vi "Parse_Ignore_string.vi"(0 "Ignore When String":string) -> (1 "Channel Name":string, 2 "Search String":string, 3 "Does Contain":bool)   [LabVIEW 2010]
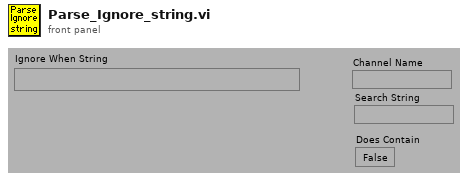
[diagram p1: front panel]
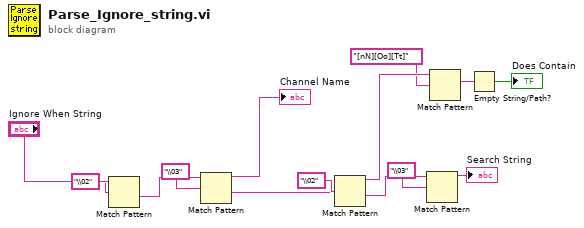
[diagram p0: block diagram]
diagram:
  n1 = Match Pattern(string="Ignore When String", regular expression="\\02") -> (after substring=w11:string)  [unwired: 4 out]
  n2 = Match Pattern(string=w11, regular expression="\\03") -> (before substring=→"Channel Name":string, after substring=w6:string)  [unwired: 3 out]
  n3 = Match Pattern(string=w6, regular expression="\\02") -> (before substring=w4:string, after substring=w9:string)  [unwired: 3 out]
  n4 = Match Pattern(string=w9, regular expression="\\03") -> (before substring=→"Search String":string)  [unwired: 4 out]
  n5 = Match Pattern(string=w4, regular expression="[nN][Oo][Tt]") -> (match substring=w2:string)  [unwired: 4 out]
  n6 = Empty String/Path?(string/path=w2) -> (empty?=→"Does Contain":bool)
